vi "S7 Read Write Cluster Array.vi"(8 "error in":errorcluster, 9 "S7 Read Write Array":T1[](array[typedef]) {"Address Areas" items=["I/O (P)"=128, "Input (I)"=129, "Output (Q)"=130, "Bit Memory (M)"=131, "Data (DB)"=132, "Instance Data (DI)"=133, "Local Data (L)"=134, "Predecessor Local Data (VL)"=135]; "Read / Write" items=["Read"=4, "Write"=5]; "Bit Number / Byte Length" max=7 step=1}, 10 "Timeout":u32, 11 "TCP Connection Ref":refnum<k5>) -> (0 "error out":errorcluster, 1 "Data Valid Array":bool[](array[boolean]), 2 "Output Data":dbl[](array[numeric]), 3 "TCP Connection Ref Out":refnum<k5>)   [LabVIEW 2011, in "S7 TCP.lvlib"]
uses:
  S7 TCP.lvlib
  S7 Read Write Cluster.ctl
  Data Type.ctl
panel:
  out "Data Read":u8[](array[numeric])
  # "Note - bits are written by first reading\nthe register byte, replacing the \ndesired bit, then writing the register\nbyte. If other bits in the register byte\nchanged durring this process will\nbe overwritten!"
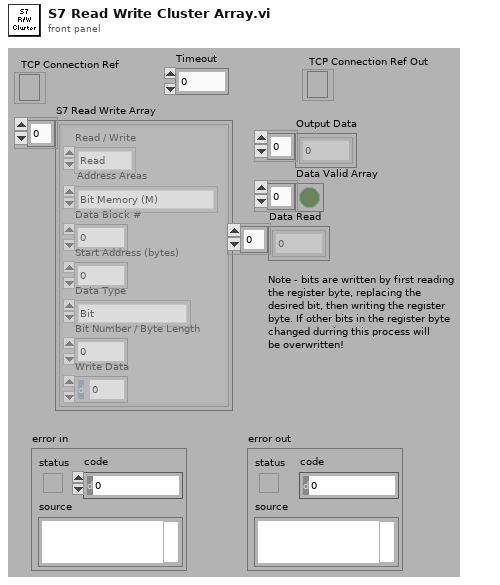
[diagram p1: front panel]
types:
  T1 = typedef "S7 TCP.lvlib/S7 Read Write Cluster.ctl" = cluster{"Read / Write":u8, "Address Areas":u8, "Data Block #":u16, "Start Address (bytes)":u32, "Data Type":T2, "Bit Number / Byte Length":u8, "Write Data":dbl}
  T2 = typedef "S7 TCP.lvlib/Data Type.ctl" = enum16{"Bit", "Byte (U8)", "Signed Byte (I8)", "Word (U16)", "Signed Word (I16)", "Long (U32)", "Signed Long (I32)", "Real (SGL)", "Defined Byte Length"}
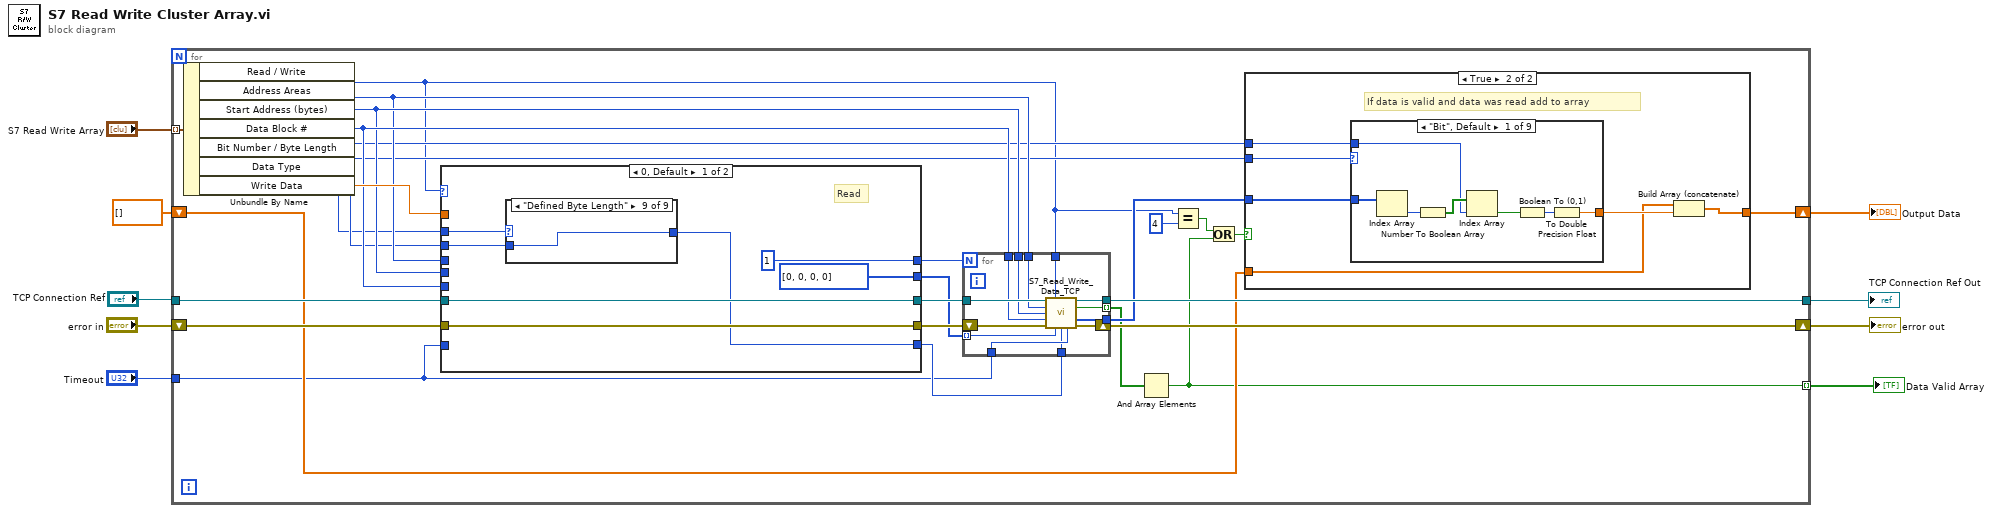
[diagram p0: block diagram]
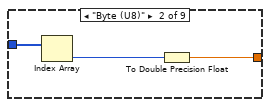
[diagram p3: hidden frame]
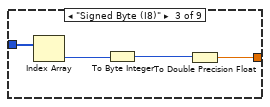
[diagram p4: hidden frame]
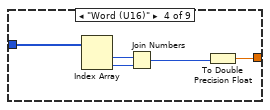
[diagram p5: hidden frame]
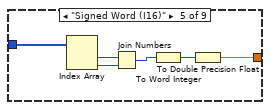
[diagram p6: hidden frame]
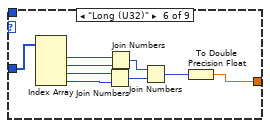
[diagram p7: hidden frame]
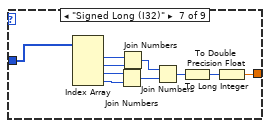
[diagram p8: hidden frame]
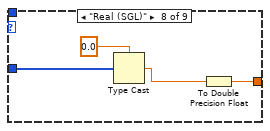
[diagram p9: hidden frame]
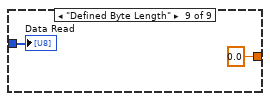
[diagram p10: hidden frame]
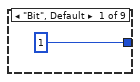
[diagram p11: hidden frame]
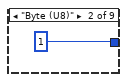
[diagram p12: hidden frame]
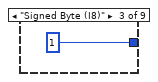
[diagram p13: hidden frame]
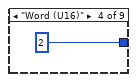
[diagram p14: hidden frame]
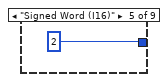
[diagram p15: hidden frame]
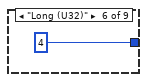
[diagram p16: hidden frame]
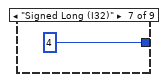
[diagram p17: hidden frame]
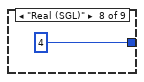
[diagram p18: hidden frame]
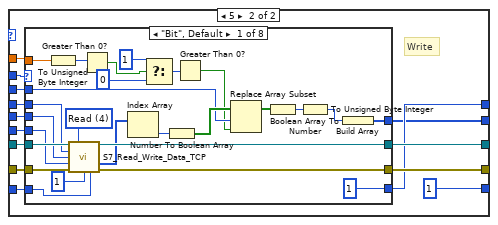
[diagram p19: hidden frame]
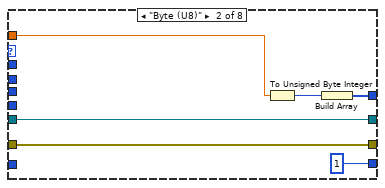
[diagram p20: hidden frame]
diagram:
  n1 = for {
    tunnel: "Timeout" -> [w10]
    tunnel: "TCP Connection Ref" -> [w29]
    tunnel: [w34] -> w1
    tunnel: "S7 Read Write Array" -> [w32] mode=indexing
    tunnel: [w16] -> w5 mode=indexing
    shift-right: [w35] -> w9
    shift-left: "error in" -> [w20]
    shift-right: [w19] -> w6
    shift-left: dbl[] [] -> [w18]
    n2 = Unbundle By Name(w32) -> ("Read / Write"=w13:u8, "Address Areas"=w24:u8, "Start Address (bytes)"=w25:u32, "Data Block #"=w26:u16, "Bit Number / Byte Length"=w23:u8, "Data Type"=w21:T2, "Write Data"=w30:dbl)
    n3 = case shown="0, Default" w13 {
      tunnel: w21 -> [w95 w122]
      tunnel: w30 -> [_ w121]
      tunnel: w29 -> [w98 w120]
      tunnel: w20 -> [w97 w119]
      tunnel: [w98 w118] -> w28
      tunnel: [w97 w117] -> w27
      tunnel: w26 -> [_ w116]
      tunnel: w25 -> [_ w115]
      tunnel: w24 -> [_ w114]
      tunnel: w23 -> [w93 w113]
      tunnel: [u8[] [0, 0, 0, 0] w109] -> w22
      tunnel: [w94 u8 1] -> w12
      tunnel: [u8 1 w112] -> w11
      tunnel: w10 -> [_ w110]
      frame 0, Default {
        # "Read"
        n4 = case shown="\"Defined Byte Length\"" w95 {
          tunnel: [u8 1 u8 1 u8 1 u8 2 u8 2 u8 4 u8 4 u8 4 w108] -> w94
          tunnel: w93 -> [_ _ _ _ _ _ _ _ w108]
          frame "Bit", Default {
          }
          frame "Byte (U8)" {
          }
          frame "Signed Byte (I8)" {
          }
          frame "Word (U16)" {
          }
          frame "Signed Word (I16)" {
          }
          frame "Long (U32)" {
          }
          frame "Signed Long (I32)" {
          }
          frame "Real (SGL)" {
          }
          frame "Defined Byte Length" {
          }
        }
      }
      frame 5 {
        # "Write"
        n5 = case shown="\"Bit\", Default" w122 {
          tunnel: w121 -> [w135 w153 w159 w169 w178 w187 w198 w208]
          tunnel: w120 -> [w148 w151 w157 w167 w175 w186 w196 w207]
          tunnel: w119 -> [w145 w150 w156 w166 w174 w185 w197 w206]
          tunnel: [w147 w151 w157 w167 w175 w186 w196 w207] -> w118
          tunnel: [w146 w150 w156 w166 w174 w185 w197 w206] -> w117
          tunnel: w116 -> [w143 _ _ _ _ _ _ _]
          tunnel: w115 -> [w142 _ _ _ _ _ _ _]
          tunnel: w114 -> [w141 _ _ _ _ _ _ _]
          tunnel: w113 -> [w136 _ _ _ _ _ _ _]
          tunnel: [w126 w152 w158 w162 w170 w179 w200 w204] -> w109
          tunnel: [u8 1 u8 1 u8 1 u8 2 u8 2 u8 4 u8 4 u8 4] -> w112
          tunnel: w110 -> [w123 _ _ _ _ _ _ _]
          frame "Bit", Default {
            w140 = u8 4 items=["Read"=4, "Write"=5] ("Read / Write")
            n6 = To Unsigned Byte Integer(number=w135) -> (unsigned 8bit integer=w132:u8)
            n7 = call "S7_Read_Write_Data_TCP.vi"("TCP Connection Ref"=w148, "Read / Write"=w140, "Address Areas"=w141, "Start Address (bytes)"=w142, "Data Block #"=w143, "error in"=w145, "Length (bytes)"=u16 1, "Timeout"=w123) -> ("TCP Connection Ref Out"=w147:refnum<k5>, "Data Read"=w139:u8[], "error out"=w146:errorcluster)  [unwired: 1 in, 4 out]
            n8 = Greater Than 0?(x=w132) -> (x > 0?=w131:bool)
            n9 = Index Array(array=w139) -> (element=w138:u8)  [unwired: 1 in]
            n10 = Select(t=1, s=w131, f=0) -> (s? t:f=w130:i32)
            n11 = Number To Boolean Array(number=w138) -> (Boolean array=w137:bool[])
            n12 = Greater Than 0?(x=w130) -> (x > 0?=w129:bool)
            n13 = Replace Array Subset(array=w137, new element=w129, index=w136) -> (w128:bool[])
            n14 = Boolean Array To Number(Boolean array=w128) -> (number=w127:u32)
            n15 = To Unsigned Byte Integer(number=w127) -> (unsigned 8bit integer=w125:u8)
            n16 = Build Array(w125) -> (w126:u8[])
          }
          frame "Byte (U8)" {
            n17 = To Unsigned Byte Integer(number=w153) -> (unsigned 8bit integer=w154:u8)
            n18 = Build Array(w154) -> (w152:u8[])
          }
          frame "Signed Byte (I8)" {
            n19 = To Byte Integer(number=w159) -> (8bit integer=w161:i8)
            n20 = To Unsigned Byte Integer(number=w161) -> (unsigned 8bit integer=w160:u8)
            n21 = Build Array(w160) -> (w158:u8[])
          }
          frame "Word (U16)" {
            n22 = To Unsigned Word Integer(number=w169) -> (unsigned 16bit integer=w168:u16)
            n23 = Split Number(x=w168) -> (hi(x)=w164:u8, lo(x)=w163:u8)
            n24 = Build Array(w164, w163) -> (w162:u8[])
          }
          frame "Signed Word (I16)" {
            n25 = To Word Integer(number=w178) -> (16bit integer=w176:i16)
            n26 = To Unsigned Word Integer(number=w176) -> (unsigned 16bit integer=w177:u16)
            n27 = Split Number(x=w177) -> (hi(x)=w171:u8, lo(x)=w172:u8)
            n28 = Build Array(w171, w172) -> (w170:u8[])
          }
          frame "Long (U32)" {
            n29 = To Unsigned Long Integer(number=w187) -> (unsigned 32bit integer=w188:u32)
            n30 = Split Number(x=w188) -> (hi(x)=w190:u16, lo(x)=w189:u16)
            n31 = Split Number(x=w190) -> (hi(x)=w183:u8, lo(x)=w182:u8)
            n32 = Split Number(x=w189) -> (hi(x)=w181:u8, lo(x)=w180:u8)
            n33 = Build Array(w183, w182, w181, w180) -> (w179:u8[])
          }
          frame "Signed Long (I32)" {
            n34 = To Long Integer(number=w198) -> (32bit integer=w199:i32)
            n35 = To Unsigned Long Integer(number=w199) -> (unsigned 32bit integer=w201:u32)
            n36 = Split Number(x=w201) -> (hi(x)=w203:u16, lo(x)=w202:u16)
            n37 = Split Number(x=w203) -> (hi(x)=w191:u8, lo(x)=w192:u8)
            n38 = Split Number(x=w202) -> (hi(x)=w193:u8, lo(x)=w194:u8)
            n39 = Build Array(w191, w192, w193, w194) -> (w200:u8[])
          }
          frame "Real (SGL)" {
            n40 = Type Cast(type=u8[] [], x=w208) -> (*(type *) &x=w204:u8[])
          }
        }
      }
    }
    n41 = for {
      N: w11 -> [_]
      tunnel: w13 -> [w222]
      tunnel: w10 -> [w220]
      tunnel: [w219] -> w34
      tunnel: [w218] -> w33
      tunnel: w12 -> [w217]
      tunnel: [w216] -> w31 mode=indexing
      tunnel: w28 -> [w215]
      tunnel: w26 -> [w213]
      tunnel: w25 -> [w212]
      tunnel: w24 -> [w211]
      tunnel: w22 -> [w210] mode=indexing
      shift-right: [w221] -> w35
      shift-left: w27 -> [w214]
      n42 = call "S7_Read_Write_Data_TCP.vi"("TCP Connection Ref"=w215, "Read / Write"=w222, "Address Areas"=w211, "Start Address (bytes)"=w212, "Data Block #"=w213, "error in"=w214, "Write Data"=w210, "Length (bytes)"=w217, "Timeout"=w220) -> ("TCP Connection Ref Out"=w219:refnum<k5>, "Data Valid"=w216:bool, "Data Read"=w218:u8[], "error out"=w221:errorcluster)  [unwired: 3 out]
    }
    n43 = And Array Elements(Boolean array=w31) -> (logical AND=w16:bool)
    n44 = Equal?(x=w13, y=u8 4) -> (x = y?=w15:bool)
    n45 = Or(x=w15, y=w16) -> (x .or. y?=w17:bool)
    n46 = case shown="True" w17 {
      tunnel: w33 -> [_ w37]
      tunnel: w23 -> [_ w41]
      tunnel: w21 -> [_ w40]
      tunnel: [w36 w39] -> w19
      tunnel: w18 -> [w36 w38]
      frame False {
      }
      frame True {
        # "If data is valid and data was read add to array"
        n47 = case shown="\"Bit\", Default" w40 {
          tunnel: w37 -> [w49 w52 w56 w61 w65 w70 w77 w90 w91]
          tunnel: w41 -> [w46 _ _ _ _ _ _ _ _]
          tunnel: [w43 w50 w55 w58 w64 w68 w80 w87 0.0] -> w42
          frame "Bit", Default {
            n48 = Index Array(array=w49) -> (element=w48:u8)  [unwired: 1 in]
            n49 = Number To Boolean Array(number=w48) -> (Boolean array=w47:bool[])
            n50 = Index Array(array=w47, index=w46) -> (element=w45:bool)
            n51 = Boolean To (0,1)(Boolean=w45) -> (0, 1=w44:i16)
            n52 = To Double Precision Float(number=w44) -> (double precision float=w43:dbl)
          }
          frame "Byte (U8)" {
            n53 = Index Array(array=w52) -> (element=w51:u8)  [unwired: 1 in]
            n54 = To Double Precision Float(number=w51) -> (double precision float=w50:dbl)
          }
          frame "Signed Byte (I8)" {
            n55 = Index Array(array=w56) -> (element=w54:u8)  [unwired: 1 in]
            n56 = To Byte Integer(number=w54) -> (8bit integer=w53:i8)
            n57 = To Double Precision Float(number=w53) -> (double precision float=w55:dbl)
          }
          frame "Word (U16)" {
            n58 = Index Array(array=w61) -> (element #1=w59:u8, element #2=w60:u8)  [unwired: 2 in]
            n59 = Join Numbers(hi=w59, lo=w60) -> ((hi.lo)=w57:u16)
            n60 = To Double Precision Float(number=w57) -> (double precision float=w58:dbl)
          }
          frame "Signed Word (I16)" {
            n61 = Index Array(array=w65) -> (element #1=w66:u8, element #2=w67:u8)  [unwired: 2 in]
            n62 = Join Numbers(hi=w66, lo=w67) -> ((hi.lo)=w63:u16)
            n63 = To Word Integer(number=w63) -> (16bit integer=w62:i16)
            n64 = To Double Precision Float(number=w62) -> (double precision float=w64:dbl)
          }
          frame "Long (U32)" {
            n65 = Index Array(array=w70) -> (element #1=w75:u8, element #2=w76:u8, element #3=w72:u8, element #4=w71:u8)  [unwired: 4 in]
            n66 = Join Numbers(hi=w72, lo=w71) -> ((hi.lo)=w73:u16)
            n67 = Join Numbers(hi=w75, lo=w76) -> ((hi.lo)=w74:u16)
            n68 = Join Numbers(hi=w74, lo=w73) -> ((hi.lo)=w69:u32)
            n69 = To Double Precision Float(number=w69) -> (double precision float=w68:dbl)
          }
          frame "Signed Long (I32)" {
            n70 = Index Array(array=w77) -> (element #1=w85:u8, element #2=w86:u8, element #3=w82:u8, element #4=w81:u8)  [unwired: 4 in]
            n71 = Join Numbers(hi=w82, lo=w81) -> ((hi.lo)=w83:u16)
            n72 = Join Numbers(hi=w85, lo=w86) -> ((hi.lo)=w84:u16)
            n73 = Join Numbers(hi=w84, lo=w83) -> ((hi.lo)=w79:u32)
            n74 = To Long Integer(number=w79) -> (32bit integer=w78:i32)
            n75 = To Double Precision Float(number=w78) -> (double precision float=w80:dbl)
          }
          frame "Real (SGL)" {
            n76 = Type Cast(type=sgl 0.0, x=w90) -> (*(type *) &x=w88:sgl)
            n77 = To Double Precision Float(number=w88) -> (double precision float=w87:dbl)
          }
          frame "Defined Byte Length" {
            "Data Read" <- w91
          }
        }
        n78 = Build Array (concatenate)(w38, w42) -> (w39:dbl[])
      }
    }
  }
  "error out" <- w9
  "Output Data" <- w6
  "Data Valid Array" <- w5
  "TCP Connection Ref Out" <- w1
